vi "Untitled 6.vi"   [LabVIEW 2020]
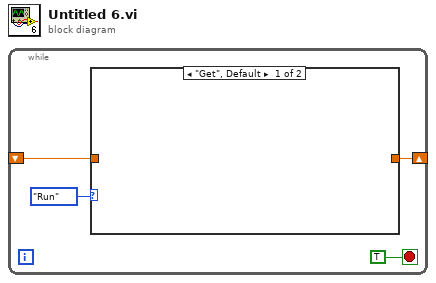
[diagram p0: block diagram]
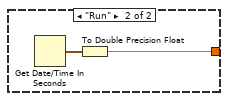
[diagram p2: hidden frame]
diagram:
  n1 = while {
    shift-right: [w4] -> _
    shift-left: _ -> [w1]
    stop <- TRUE stop-if-true
    n2 = case shown="\"Get\", Default" enum16{"Get", "Run"}."Run" {
      tunnel: [_ w5] -> w4
      tunnel: w1 -> [_ _]
      frame "Get", Default {
      }
      frame "Run" {
        n3 = Get Date/Time In Seconds() -> (seconds since 1Jan1904=w6:timestamp)
        n4 = To Double Precision Float(number=w6) -> (double precision float=w5:dbl)
      }
    }
  }
